vi "Elapsed Timer.vi"(8 "error in":errorcluster, 11 "reset":bool) -> (0 "error out":errorcluster, 2 "since last call":u32, 3 "elapsed time":u32)   [LabVIEW 2013, in "毫秒定时器.lvlib"]
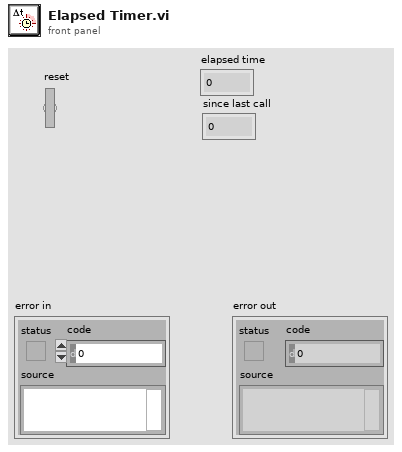
[diagram p1: front panel]
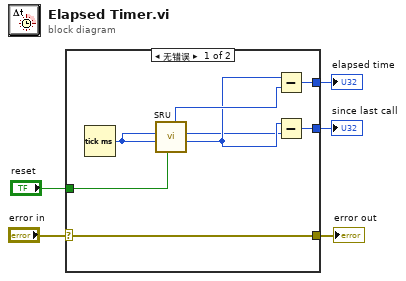
[diagram p0: block diagram]
diagram:
  n1 = case shown="无错误" "error in" {
    selector: "error in" -> [w13 w14]
    tunnel: [w13 w14] -> w5
    tunnel: "reset" -> [w8 _]
    tunnel: [w7 _] -> w2
    tunnel: [w6 _] -> w1
    frame No Error {
      n2 = Tick Count (ms)() -> (millisecond timer value=w12:u32)
      n3 = call-poly "SRU.vi"("复位"=w8, "初始值"=w12, "输入"=w12) -> ("本次值"=w10:u32, "上次值"=w9:u32, "初始值"=w11:u32)  [unwired: 6 in]
      n4 = Subtract(x=w10, y=w11) -> (x-y=w7:u32)
      n5 = Subtract(x=w10, y=w9) -> (x-y=w6:u32)
    }
    frame Error {
    }
  }
  "error out" <- w5
  "elapsed time" <- w2
  "since last call" <- w1
